vi "Hella BLDC Seed 2 Key.vi"(8 "MSG 2":u8[](array[numeric])=[33, 251, 203, 47, 36, 170, 170, 170] format="%.0x", 11 "MSG 1":u8[](array[numeric])=[16, 10, 103, 55, 251, 203, 47, 36] format="%.0x") -> (3 "Security Response":u8[](array[numeric]) format="%.0x")   [LabVIEW 2013]
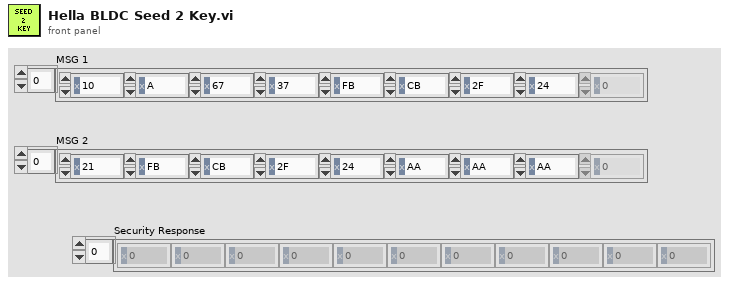
[diagram p1: front panel]
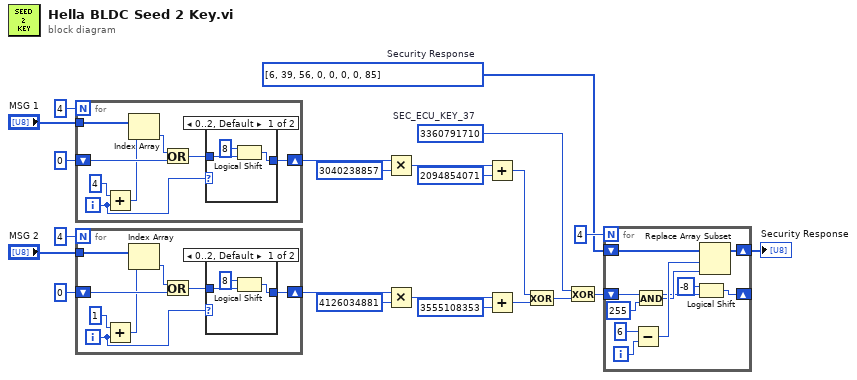
[diagram p0: block diagram]
diagram:
  w3 = u8[] [6, 39, 56, 0, 0, 0, 0, 85]  # Security Response
  w20 = u32 3360791710  # SEC_ECU_KEY_37
  n1 = for {
    N: 4 -> [_]
    tunnel: "MSG 1" -> [w28]
    shift-right: [w24] -> w10
    shift-left: u32 0 -> [w29]
    i -> [w23]
    n2 = Add(x=4, y=w23) -> (x+y=w27:i32)
    n3 = Index Array(array=w28, index=w27) -> (element=w26:u8)
    n4 = Or(x=w26, y=w29) -> (x .or. y?=w25:u32)
    n5 = case shown="0..2, Default" w23 {
      tunnel: w25 -> [w33 w34]
      tunnel: [w31 w34] -> w24
      frame 0..2, Default {
        n6 = Logical Shift(y=i16 8, x=w33) -> (x << y=w31:u32)
      }
      frame 3 {
      }
    }
  }
  n7 = for {
    N: 4 -> [_]
    tunnel: "MSG 2" -> [w40]
    shift-right: [w36] -> w17
    shift-left: u32 0 -> [w41]
    i -> [w35]
    n8 = Add(x=1, y=w35) -> (x+y=w39:i32)
    n9 = Index Array(array=w40, index=w39) -> (element=w38:u8)
    n10 = Or(x=w38, y=w41) -> (x .or. y?=w37:u32)
    n11 = case shown="0..2, Default" w35 {
      tunnel: w37 -> [w45 w46]
      tunnel: [w43 w46] -> w36
      frame 0..2, Default {
        n12 = Logical Shift(y=i16 8, x=w45) -> (x << y=w43:u32)
      }
      frame 3 {
      }
    }
  }
  n13 = Multiply(x=w10, y=u32 3040238857) -> (x*y=w11:u32)
  n14 = Multiply(x=w17, y=u32 4126034881) -> (x*y=w16:u32)
  n15 = Add(x=w11, y=u32 2094854071) -> (x+y=w18:u32)
  n16 = Add(x=w16, y=u32 3555108353) -> (x+y=w19:u32)
  n17 = Exclusive Or(1:w19, 2:w18) -> (0:w21:u32)
  n18 = Exclusive Or(1:w21, 2:w20) -> (0:w2:u32)
  n19 = for {
    N: 4 -> [_]
    shift-right: [w55] -> w1
    shift-left: w3 -> [w56]
    shift-right: [w48] -> _
    shift-left: w2 -> [w49]
    i -> [w54]
    n20 = Subtract(x=6, y=w54) -> (x-y=w52:i32)
    n21 = And(x=w49, y=u32 255) -> (x .and. y?=w50:u32)
    n22 = Logical Shift(y=i16 -8, x=w49) -> (x << y=w48:u32)
    n23 = Replace Array Subset(array=w56, new element=w50, index=w52) -> (w55:u8[])
  }
  "Security Response" <- w1
